vi "sub_conv_dec.vi"(6 "code type":T1(ring), 7 "decision type":enum16{"hard decision", "soft decision"}(ring), 8 "output in decimal":u32[][](array[numeric]), 9 "state transition":u32[][](array[numeric]), 10 "symbol map":cdb[](array[numeric]), 11 "hard bits/soft symbols":cdb[](array[numeric])) -> (3 "Decoded":bool[](array[boolean]))   [LabVIEW 2014]
panel:
  out "Array 2":dbl[][](array[numeric])
  out "Array":i32[][](array[numeric])
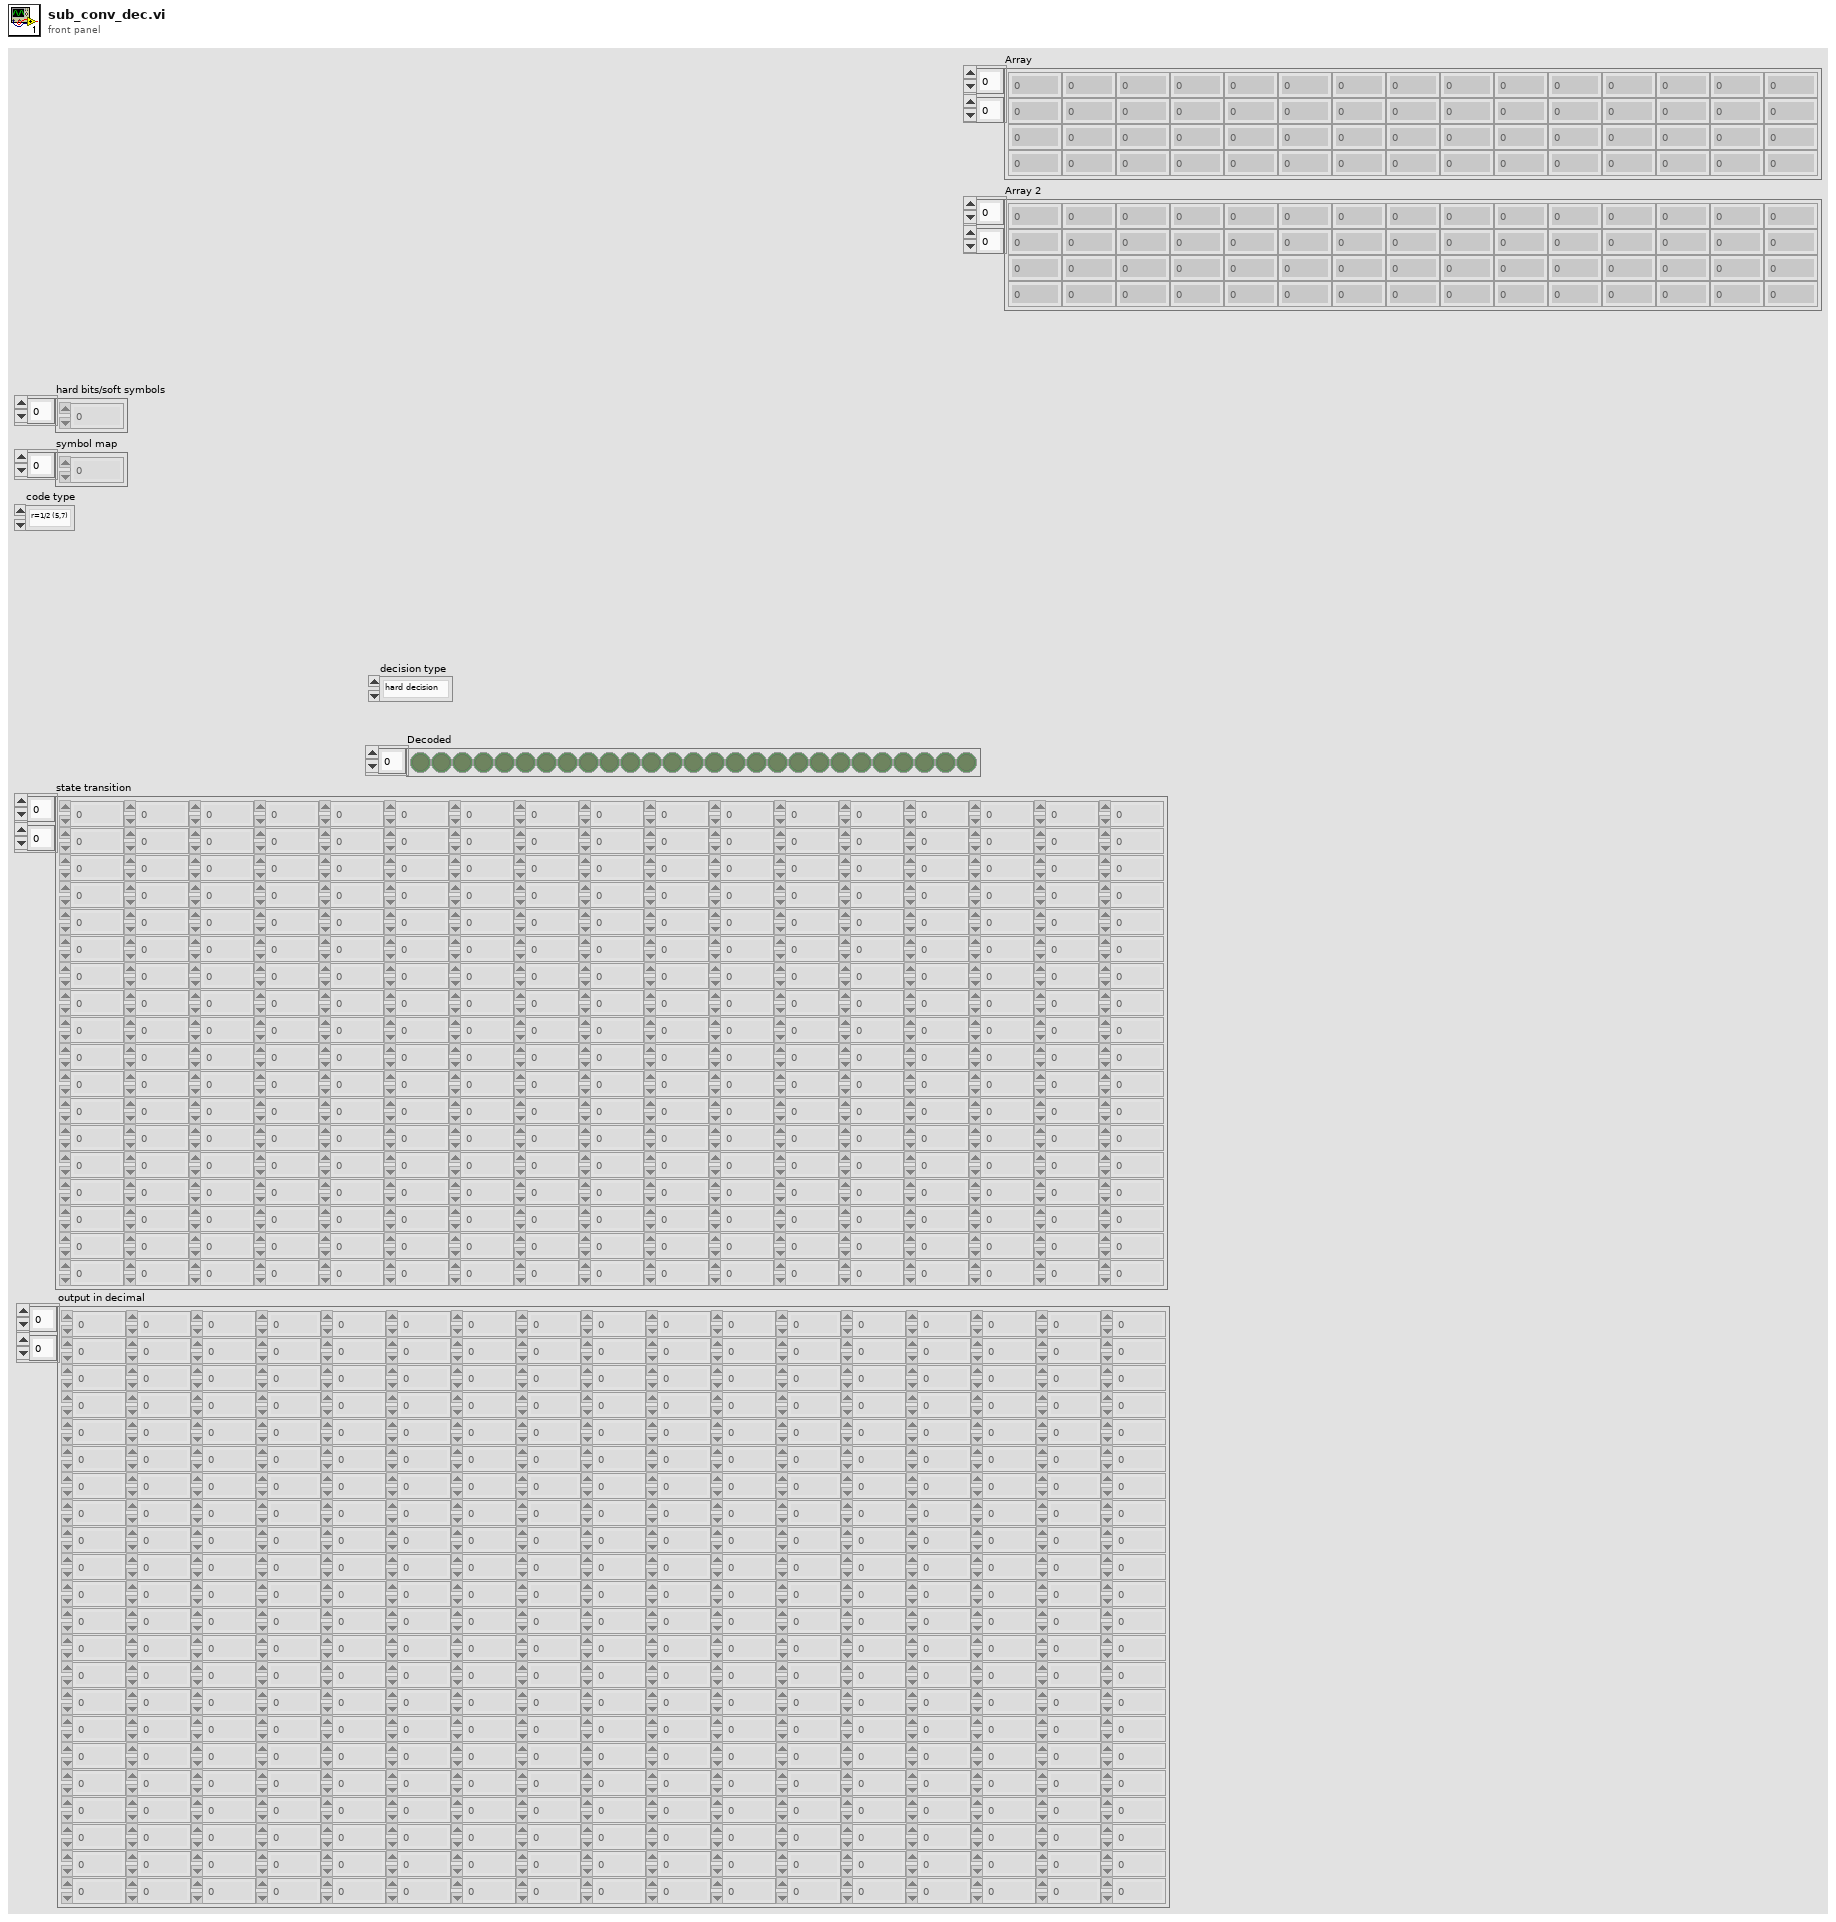
[diagram p1: front panel]
types:
  T1 = enum16{"r=1/2 (5,7)", "r=1/2 (13,17)", "r=1/4 (25,27,33,37)"}
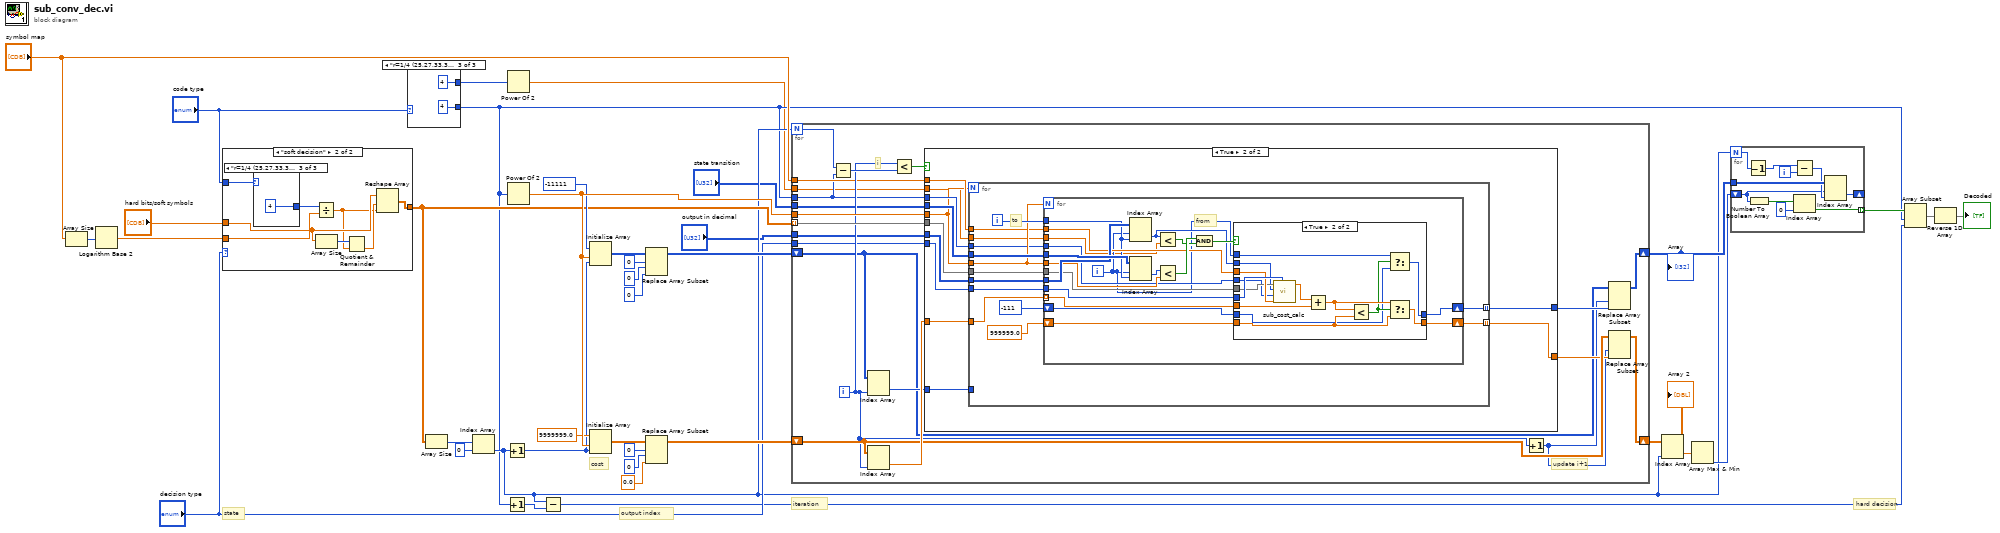
[diagram p0: block diagram]
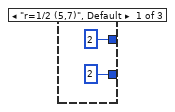
[diagram p2: hidden frame]
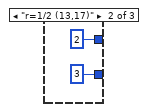
[diagram p3: hidden frame]
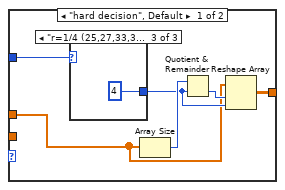
[diagram p4: hidden frame]
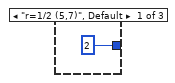
[diagram p5: hidden frame]
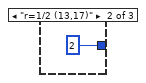
[diagram p6: hidden frame]
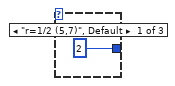
[diagram p7: hidden frame]
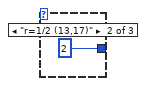
[diagram p8: hidden frame]
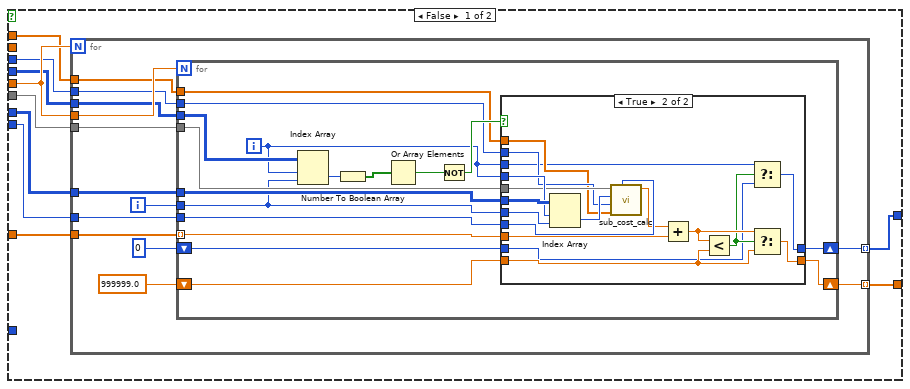
[diagram p9: hidden frame]
diagram:
  # "output index"
  # "state"
  # "cost"
  # "iteration"
  # "hard decision"
  n1 = Array Size(array="symbol map") -> (size(s)=w38:i32)
  n2 = Logarithm Base 2(1:w38) -> (0:w37:dbl)
  n3 = case shown="\"soft decision\"" "decision type" {
    tunnel: "hard bits/soft symbols" -> [w39 w52]
    tunnel: "code type" -> [w44 w55]
    tunnel: w37 -> [_ w53]
    tunnel: [w40 w48] -> w23
    frame "hard decision", Default {
      n4 = case shown="\"r=1/4 (25,27,33,37)\"" w44 {
        tunnel: [2 2 4] -> w41
        frame "r=1/2 (5,7)", Default {
        }
        frame "r=1/2 (13,17)" {
        }
        frame "r=1/4 (25,27,33,37)" {
        }
      }
      n5 = Array Size(array=w39) -> (size(s)=w43:i32)
      n6 = Quotient & Remainder(x=w43, y=w41) -> (floor(x/y)=w42:i32)  [unwired: 1 out]
      n7 = Reshape Array(w39, w42, w41) -> (w40:cdb[][])
    }
    frame "soft decision" {
      n8 = case shown="\"r=1/4 (25,27,33,37)\"" w55 {
        tunnel: [2 2 4] -> w54
        frame "r=1/2 (5,7)", Default {
        }
        frame "r=1/2 (13,17)" {
        }
        frame "r=1/4 (25,27,33,37)" {
        }
      }
      n9 = Divide(x=w54, y=w53) -> (x/y=w49:dbl)
      n10 = Array Size(array=w52) -> (size(s)=w51:i32)
      n11 = Quotient & Remainder(x=w51, y=w49) -> (floor(x/y)=w50:dbl)  [unwired: 1 out]
      n12 = Reshape Array(w52, w50, w49) -> (w48:cdb[][])
    }
  }
  n13 = case shown="\"r=1/4 (25,27,33,37)\"" "code type" {
    tunnel: [2 3 4] -> w5
    tunnel: [2 2 4] -> w2
    frame "r=1/2 (5,7)", Default {
    }
    frame "r=1/2 (13,17)" {
    }
    frame "r=1/4 (25,27,33,37)" {
    }
  }
  n14 = Array Size(array=w23) -> (size(s)=w28:i32[])
  n15 = Index Array(array=w28, index=0) -> (element=w9:i32)
  n16 = Increment(x=w9) -> (x+1=w24:i32)
  n17 = Increment(x=w5) -> (x+1=w8:i32)
  n18 = Power Of 2(x=w2) -> (2^x=w1:dbl)
  n19 = Power Of 2(x=w5) -> (2^x=w36:dbl)
  n20 = Subtract(x=w9, y=w8) -> (x-y=w7:i32)
  n21 = Initialize Array(-11111, w36, w24) -> (w17:i32[][])
  n22 = Initialize Array(9999999.0, w36, w24) -> (w22:dbl[][])
  n23 = Replace Array Subset(array=w17, new element=0 ("new element/subarray"), index (row)=0, index (col)=0 ("disabled index (col)")) -> (w13:i32[][])
  n24 = Replace Array Subset(array=w22, new element=0.0 ("new element/subarray"), index (row)=0, index (col)=0 ("disabled index (col)")) -> (w18:dbl[][])
  n25 = for {
    N: w9 -> [w83]
    shift-right: [w72] -> w35
    shift-left: w18 -> [w79]
    tunnel: w23 -> [w84] mode=indexing
    tunnel: w36 -> [w85]
    shift-right: [w73] -> w33
    shift-left: w13 -> [w75]
    tunnel: w5 -> [w67]
    tunnel: "state transition" -> [w71]
    tunnel: "output in decimal" -> [w70]
    tunnel: "decision type" -> [w69]
    tunnel: "symbol map" -> [w68]
    tunnel: w1 -> [w65]
    i -> [w78]
    # "update i+1"
    # "i"
    n26 = Subtract(x=w83, y=w67) -> (x-y=w82:i32)
    n27 = Index Array(array=w75, index (col)=w78) -> (element=w80:i32[])  [unwired: 1 in]
    n28 = Index Array(array=w79, index (col)=w78) -> (element=w81:dbl[])  [unwired: 1 in]
    n29 = Less?(x=w78, y=w82) -> (x < y?=w66:bool)
    n30 = case shown="True" w66 {
      tunnel: w85 -> [w95 w146]
      tunnel: w84 -> [w92 w156]
      tunnel: w81 -> [w88 w155]
      tunnel: w80 -> [_ w154]
      tunnel: [w87 w153] -> w77
      tunnel: [w86 w152] -> w76
      tunnel: w71 -> [w94 w151]
      tunnel: w70 -> [w93 w150]
      tunnel: w69 -> [w89 w149]
      tunnel: w68 -> [w90 w148]
      tunnel: w67 -> [w91 w147]
      tunnel: w65 -> [_ w145]
      frame False {
        n31 = for {
          N: w95 -> [_]
          tunnel: w95 -> [w108]
          tunnel: w94 -> [w107]
          tunnel: w93 -> [w105]
          tunnel: w92 -> [w104]
          tunnel: w91 -> [w103]
          tunnel: w90 -> [w102]
          tunnel: w89 -> [w101]
          tunnel: w88 -> [w100]
          tunnel: [w97] -> w87 mode=indexing
          tunnel: [w96] -> w86 mode=indexing
          i -> [w106]
          n32 = for {
            N: w108 -> [_]
            tunnel: w107 -> [w125]
            tunnel: w106 -> [w110]
            tunnel: w105 -> [w120]
            tunnel: w104 -> [w119]
            tunnel: w103 -> [w118]
            tunnel: w102 -> [w117]
            tunnel: w101 -> [w116]
            tunnel: w100 -> [w115] mode=indexing
            shift-right: [w113] -> w97
            shift-left: 999999.0 -> [w114]
            shift-right: [w111] -> w96
            shift-left: 0 -> [w112]
            i -> [w109]
            n33 = Index Array(array=w125, index (row)=w109, index (col)=w110) -> (element=w124:u32)
            n34 = Number To Boolean Array(number=w124) -> (Boolean array=w123:bool[])
            n35 = Or Array Elements(Boolean array=w123) -> (logical OR=w122:bool)
            n36 = Not(x=w122) -> (.not. x?=w121:bool)
            n37 = case shown="True" w121 {
              tunnel: w120 -> [_ w144]
              tunnel: w109 -> [_ w143]
              tunnel: w110 -> [_ w142]
              tunnel: w119 -> [_ w140]
              tunnel: w118 -> [_ w139]
              tunnel: w117 -> [_ w138]
              tunnel: w116 -> [_ w137]
              tunnel: w115 -> [_ w136]
              tunnel: w114 -> [w126 w133]
              tunnel: [w126 w132] -> w113
              tunnel: w112 -> [w127 w129]
              tunnel: w109 -> [_ w128]
              tunnel: [w127 w130] -> w111
              frame False {
              }
              frame True {
                n38 = Index Array(array=w144, index (row)=w143, index (col)=w142) -> (element=w141:u32)
                n39 = call "sub_cost_calc.vi"("decision type"=w137, "symbol map"=w138, "m"=w139, "output bits in decimal"=w141, "soft symbols/ hard bits"=w140) -> ("cost function"=w135:dbl)  [unwired: 6 in]
                n40 = Add(x=w135, y=w136) -> (x+y=w134:dbl)
                n41 = Less?(x=w134, y=w133) -> (x < y?=w131:bool)
                n42 = Select(t=w128, s=w131, f=w129) -> (s? t:f=w130:i32)
                n43 = Select(t=w134, s=w131, f=w133) -> (s? t:f=w132:dbl)
              }
            }
          }
        }
      }
      frame True {
        n44 = for {
          N: w146 -> [_]
          tunnel: w156 -> [w164]
          tunnel: w155 -> [w162]
          tunnel: w154 -> [_]
          tunnel: [w159] -> w153 mode=indexing
          tunnel: [w158] -> w152 mode=indexing
          tunnel: w151 -> [w169]
          tunnel: w150 -> [w167]
          tunnel: w149 -> [w166]
          tunnel: w148 -> [w165]
          tunnel: w147 -> [w163]
          tunnel: w146 -> [w168]
          tunnel: w145 -> [w157]
          i -> [w170]
          # "to"
          n45 = for {
            N: w168 -> [_]
            tunnel: w170 -> [w173]
            tunnel: w169 -> [w190]
            tunnel: w168 -> [w187]
            tunnel: w167 -> [w188]
            tunnel: w166 -> [w183]
            tunnel: w165 -> [w182]
            tunnel: w164 -> [w181]
            tunnel: w163 -> [w180]
            tunnel: w162 -> [w178] mode=indexing
            shift-right: [w174] -> w158
            shift-left: -111 -> [w175]
            shift-right: [w176] -> w159
            shift-left: 999999.0 -> [w177]
            tunnel: w157 -> [w171]
            i -> [w172]
            # "from"
            n46 = Index Array(array=w188, index (row)=w172, index (col)=w173) -> (element=w179:u32)
            n47 = Index Array(array=w190, index (row)=w172, index (col)=w173) -> (element=w189:u32)
            n48 = Less?(x=w179, y=w171) -> (x < y?=w185:bool)
            n49 = Less?(x=w189, y=w187) -> (x < y?=w186:bool)
            n50 = And(x=w186, y=w185) -> (x .and. y?=w184:bool)
            n51 = case shown="True" w184 {
              tunnel: w183 -> [_ w206]
              tunnel: w182 -> [_ w205]
              tunnel: w181 -> [_ w204]
              tunnel: w180 -> [_ w203]
              tunnel: w179 -> [_ w202]
              tunnel: w178 -> [_ w200]
              tunnel: w177 -> [w192 w198]
              tunnel: [w192 w197] -> w176
              tunnel: w175 -> [w191 w195]
              tunnel: w172 -> [_ w194]
              tunnel: [w191 w193] -> w174
              frame False {
              }
              frame True {
                n52 = call "sub_cost_calc.vi"("decision type"=w206, "symbol map"=w205, "m"=w203, "output bits in decimal"=w202, "soft symbols/ hard bits"=w204) -> ("cost function"=w201:dbl)  [unwired: 6 in]
                n53 = Add(x=w201, y=w200) -> (x+y=w199:dbl)
                n54 = Less?(x=w199, y=w198) -> (x < y?=w196:bool)
                n55 = Select(t=w194, s=w196, f=w195) -> (s? t:f=w193:i32)
                n56 = Select(t=w199, s=w196, f=w198) -> (s? t:f=w197:dbl)
              }
            }
          }
        }
      }
    }
    n57 = Increment(x=w78) -> (x+1=w74:i32)
    n58 = Replace Array Subset(array=w75, new element=w76, index (col)=w74) -> (w73:i32[][])  [unwired: 1 in]
    n59 = Replace Array Subset(array=w79, new element=w77, index (col)=w74) -> (w72:dbl[][])  [unwired: 1 in]
  }
  "Array" <- w33
  "Array 2" <- w35
  n60 = Index Array(array=w35, index (col)=w9) -> (element=w34:dbl[])  [unwired: 1 in]
  n61 = Array Max & Min(array=w34) -> (min index (indices)=w32:i32)  [unwired: 3 out]
  n62 = for {
    N: w9 -> [w215]
    tunnel: w33 -> [w216]
    shift-right: [w211] -> _
    shift-left: w32 -> [w210]
    tunnel: [w207] -> w30 mode=indexing
    i -> [w213]
    n63 = Decrement(x=w215) -> (x-1=w214:i32)
    n64 = Number To Boolean Array(number=w210) -> (Boolean array=w209:bool[])
    n65 = Subtract(x=w214, y=w213) -> (x-y=w212:i32)
    n66 = Index Array(array=w209, index=0) -> (element=w207:bool)
    n67 = Index Array(array=w216, index (row)=w210, index (col)=w212) -> (element=w211:i32)
  }
  n68 = Array Subset(array=w30, index=w5, length=w7) -> (w29:bool[])
  n69 = Reverse 1D Array(array=w29) -> (reversed array=→"Decoded":bool[])
